vi "MCL - Set Row Background Colour.vi"(8 "Error In":errorcluster, 9 "Row Background Colour":u32(colorbox)=13158600, 10 "Row index":i32, 11 "MCL Reference":refnum<vi>) -> (0 "Error Out":errorcluster)   [LabVIEW 2023, in "Error Manager.lvlib"]
doc: "Blank VI with error handling."
uses:
  Error Manager.lvlib
  <vilib>/Utility/miscctls.llb/LVRowAndColumnTypeDef.ctl
panel:
  # "Input\nInputs to the VI"
  # "Development\nControls or indicators that are useful for development or testing, but which are not outputs of the VI."
  # "Output\nOutputs of the VI"
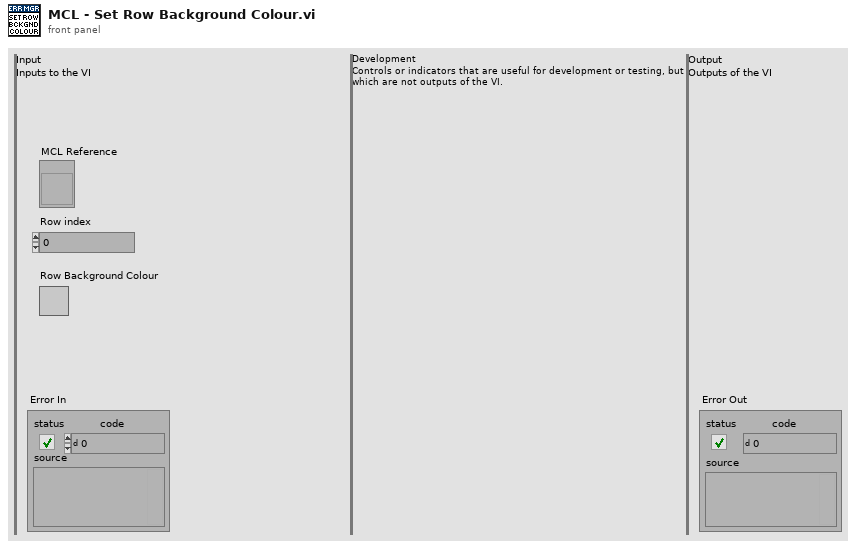
[diagram p1: front panel]
types:
  T1 = typedef "LVRowAndColumnTypeDef.ctl" = cluster{"Row":i32, "Column":i32}
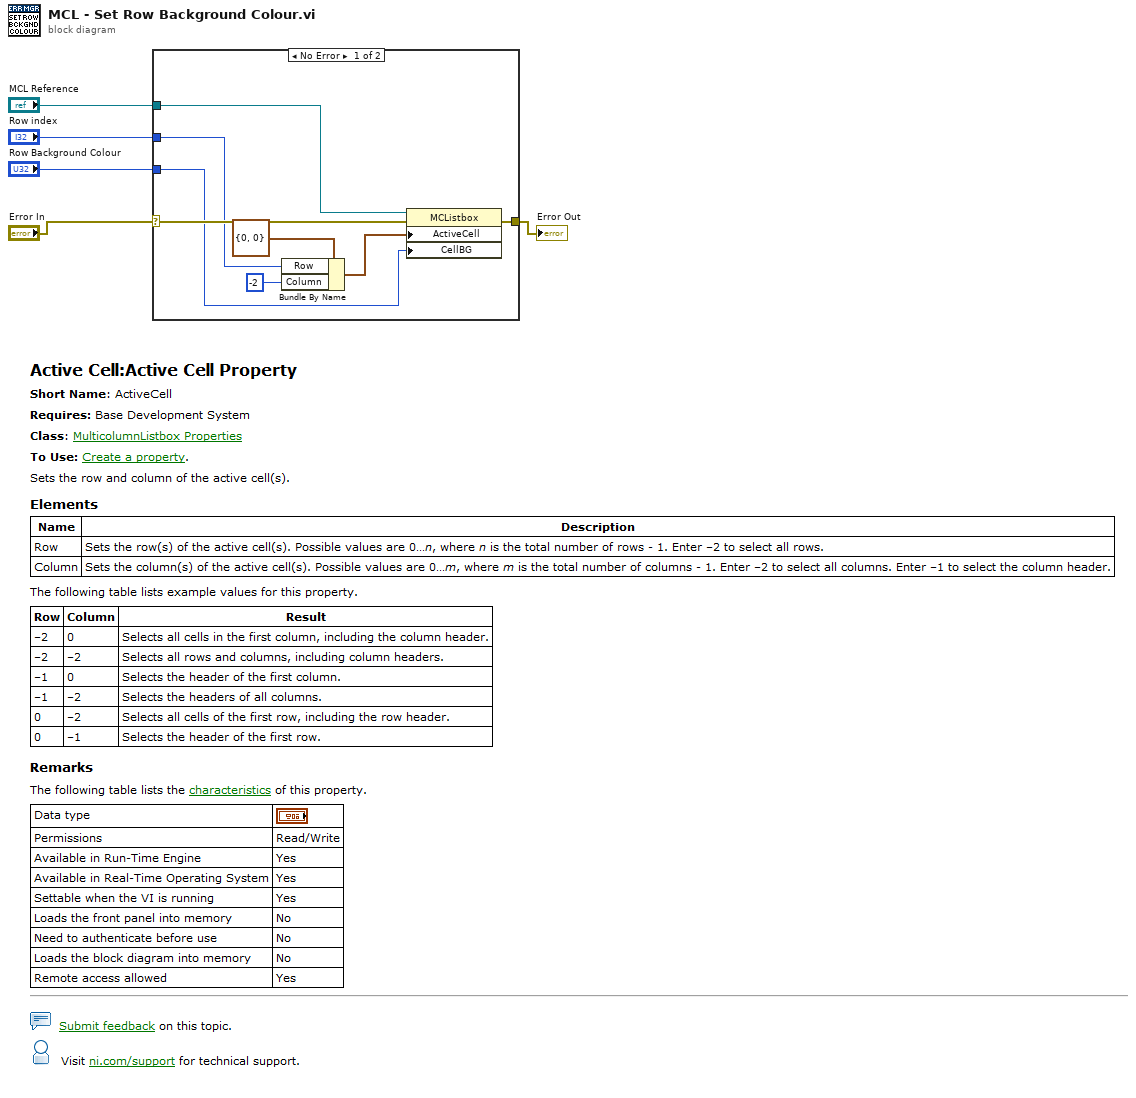
[diagram p0: block diagram]
diagram:
  n1 = case shown="No Error" "Error In" {
    selector: "Error In" -> [w13 w14]
    tunnel: [w12 w14] -> w4
    tunnel: "MCL Reference" -> [w11 _]
    tunnel: "Row index" -> [w9 _]
    tunnel: "Row Background Colour" -> [w6 _]
    frame No Error {
      n2 = Bundle By Name(cluster=T1 {"Row"=0, "Column"=0} ("Active Cell:Active Cell"), "Row"=w9, "Column"=-2) -> (w7:T1)
      n3 = property class="MCListbox"(reference=w11, error in=w13, "ActiveCell"=w7, "CellBG"=w6) -> (error out=w12:errorcluster)  [unwired: 1 out]
    }
    frame Error {
    }
  }
  "Error Out" <- w4
